vi "I2C loopback.vi"() -> ()   [LabVIEW 8.6]
uses:
  <libdir>/resource/objmgr/UeiDaq.rc
  <vilib>/UeiDaq/UeiDaqCreateI2CMasterSession.vi
  <vilib>/UeiDaq/UeiDaqConfigureTimingForMessagingIO.vi
  <vilib>/UeiDaq/UeiDaqCreateI2CSlaveSession.vi
panel:
  in  "Message Size":i32
  out "Slave Read Data String":string
  out "Master Read Data String":string
  out "Slave Read Count":i32
  out "Master Read Count":i32
  out "Command Type":u32(ring) items=["Write", "Read", "WriteRead"]
  out "Slave Tx Data":u16[](array[numeric]) format="%x"
  out "Slave Channel":i32
  out "Master Channel":i32
  in  "Stop":bool
  in  "Slave Address":i32 format="%x"
  in  "Slave Address Width":i32(ring) items=["7-bit", "10-bit"]
  in  "Bit Rate":i32(ring) items=["100kBitsPerSecond", "400kBitsPerSecond", "1MBitsPerSecond"]
  in  "TTL Level":i32(ring) items=["3.3V", "5V"]
  in  "Secure Shell?":bool
  out "Device Name":string
  in  "Resource":string
  # "I2C Loopback"
  # "Master and Slave\nCommon Configuration"
  # "Master Specific Configuration"
  # "Slave Specific Configuration"
  # "Device info"
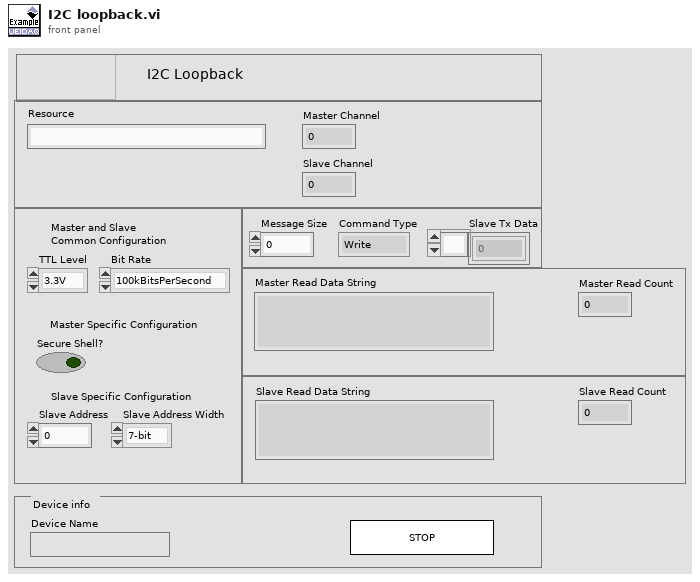
[diagram p1: front panel]
types:
  T1 = cluster{"Command":u32, "Slave Address":i32, "Slave Address Width":u32, "Number Elements to Write":i32, "Number Elements to Read":i32, "Write Data":u8[]}
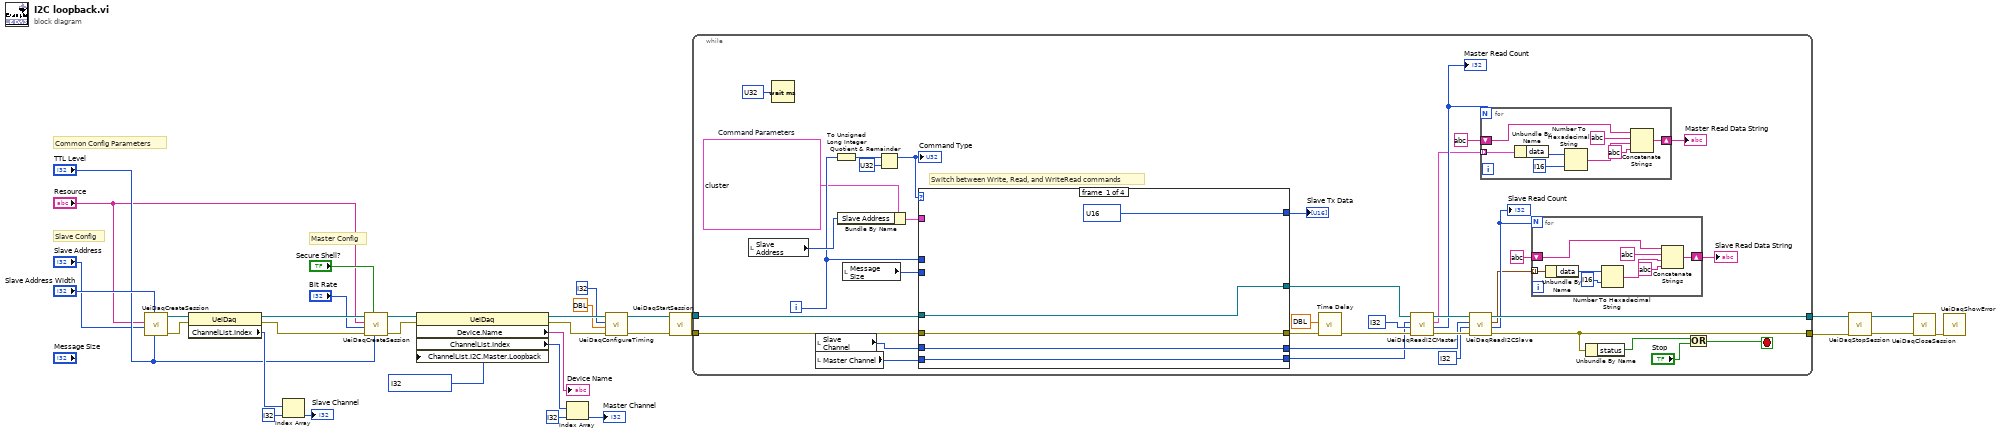
[diagram p0: block diagram]
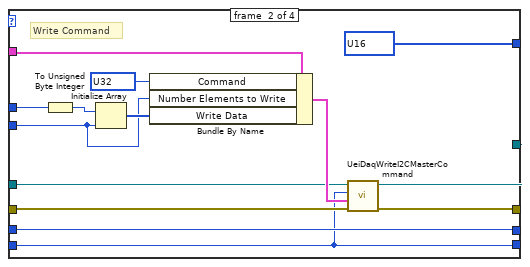
[diagram p2: hidden frame]
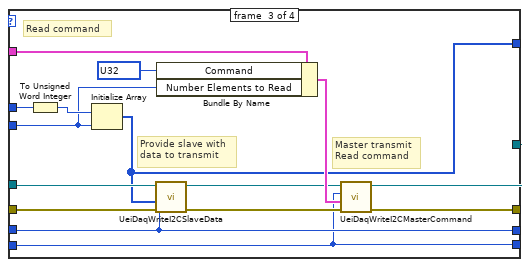
[diagram p3: hidden frame]
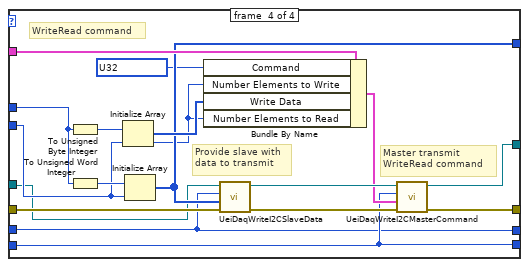
[diagram p4: hidden frame]
diagram:
  w5 = i32[] ? items=["None", "Relay", "FPGA"] ("Channel List:I2C:Master:Loopback")
  # "Master Config"
  # "Slave Config"
  # "Common Config Parameters"
  n1 = call-poly <vilib>:"UeiDaqCreateSession.vi"("TTL Level"="TTL Level", "Slave Address Width"="Slave Address Width", "Slave Address"="Slave Address", "Resource"="Resource") -> ("error out"=w22:errorcluster, "UeiDaq Refnum Out"=w25:refnum<k20>)  [unwired: 6 in]
  n2 = property class="UeiDaq"(reference=w25, error in=w22) -> (reference out=w32:refnum<k20>, error out=w31:errorcluster, "ChannelList.Index"=w27:i32[])
  n3 = Index Array(array=w27, index=i32 ?) -> (element=→"Slave Channel":i32)
  n4 = call-poly <vilib>:"UeiDaqCreateSession.vi"("TTL Level"="TTL Level", "Enable Secure Shell"="Secure Shell?", "error in (no error)"=w31, "Bit Rate"="Bit Rate", "Resource"="Resource", "UeiDaq Refnum In"=w32) -> ("error out"=w24:errorcluster, "UeiDaq Refnum Out"=w23:refnum<k20>)  [unwired: 4 in]
  n5 = property class="UeiDaq"(reference=w23, error in=w24, "ChannelList.I2C.Master.Loopback"=w5) -> (reference out=w12:refnum<k20>, error out=w11:errorcluster, "Device.Name"=→"Device Name":string, "ChannelList.Index"=w26:i32[])
  n6 = Index Array(array=w26, index=i32 ?) -> (element=→"Master Channel":i32)
  n7 = call-poly <vilib>:"UeiDaqConfigureTiming.vi"("error in (no error)"=w11, "Refresh rate"=dbl ?, "bufferSize"=i32 ?, "UeiDaq Refnum In"=w12) -> ("error out"=w16:errorcluster, "UeiDaq Refnum Out"=w15:refnum<k20>)  [unwired: 6 in]
  n8 = call <vilib>:"UeiDaqStartSession.vi"("error in (no error)"=w16, "UeiDaq Refnum In"=w15) -> ("error out"=w14:errorcluster, "UeiDaq Refnum Out"=w13:refnum<k20>)  [unwired: 8 in]
  n9 = while {
    tunnel: w14 -> [w68]
    tunnel: w13 -> [w67]
    tunnel: [w60] -> w9
    tunnel: [w51] -> w8
    i -> [w39]
    stop <- w37 stop-if-true
    w34 = T1 ?  # Command Parameters
    # "Switch between Write, Read, and WriteRead commands"
    n10 = local read "Slave Address"() -> (w55:i32)
    n11 = Wait (ms)(milliseconds to wait=u32 ?) -> ()  [unwired: 1 out]
    n12 = local read "Slave Channel"() -> (w43:i32)
    n13 = local read "Master Channel"() -> (w38:i32)
    n14 = To Unsigned Long Integer(number=w39) -> (unsigned 32bit integer=w63:u32)
    n15 = Bundle By Name(cluster=w34, "Slave Address"=w55) -> (w56:T1)
    n16 = local read "Message Size"() -> (w44:i32)
    n17 = Quotient & Remainder(x=w63, y=u32 ?) -> (x-y*floor(x/y)=w40:u32)  [unwired: 1 out]
    "Command Type" <- w40
    n18 = case shown="0" w40 {
      tunnel: w68 -> [w91 w100 w120 w134]
      tunnel: w67 -> [w90 w101 w119 w122]
      tunnel: w39 -> [_ w103 w114 w135]
      tunnel: w56 -> [_ w93 w108 w133]
      tunnel: [w90 w98 w116 w131] -> w66
      tunnel: [w91 w99 w111 w130] -> w53
      tunnel: [u16[] ? u16[] ? w107 w127] -> w62
      tunnel: w44 -> [_ w96 w106 w126]
      tunnel: w43 -> [w88 w95 w110 w123]
      tunnel: w38 -> [w87 w94 w109 w125]
      tunnel: [w88 w95 w110 w123] -> w42
      tunnel: [w87 w94 w109 w125] -> w41
      frame #0 {
      }
      frame #1 {
        w105 = u32 ? items=["Write", "Read", "WriteRead"] ("Command")
        # "Write Command"
        n19 = To Unsigned Byte Integer(number=w103) -> (unsigned 8bit integer=w92:u8)
        n20 = Initialize Array(w92, w96) -> (w104:u8[])
        n21 = Bundle By Name(cluster=w93, "Command"=w105, "Number Elements to Write"=w96, "Write Data"=w104) -> (w102:T1)
        n22 = call <vilib>:"UeiDaqWriteI2CMasterCommand.vi"("error in (no error)"=w100, "Command"=w102, "Port"=w94, "UeiDaq Refnum In"=w101) -> ("error out"=w99:errorcluster, "UeiDaq Refnum Out"=w98:refnum<k20>)  [unwired: 6 in]
      }
      frame #2 {
        w115 = u32 ? items=["Write", "Read", "WriteRead"] ("Command")
        # "Master transmit\nRead command"
        # "Provide slave with\ndata to transmit"
        # "Read command"
        n23 = To Unsigned Word Integer(number=w114) -> (unsigned 16bit integer=w113:u16)
        n24 = Initialize Array(w113, w106) -> (w107:u16[])
        n25 = call <vilib>:"UeiDaqWriteI2CSlaveData.vi"("error in (no error)"=w120, "Data"=w107, "Port"=w110, "UeiDaq Refnum In"=w119) -> ("error out"=w112:errorcluster, "UeiDaq Refnum Out"=w117:refnum<k20>)  [unwired: 5 in, 1 out]
        n26 = Bundle By Name(cluster=w108, "Command"=w115, "Number Elements to Read"=w106) -> (w118:T1)
        n27 = call <vilib>:"UeiDaqWriteI2CMasterCommand.vi"("error in (no error)"=w112, "Command"=w118, "Port"=w109, "UeiDaq Refnum In"=w117) -> ("error out"=w111:errorcluster, "UeiDaq Refnum Out"=w116:refnum<k20>)  [unwired: 6 in]
      }
      frame #3 {
        w121 = u32 ? items=["Write", "Read", "WriteRead"] ("Command")
        # "Master transmit\nWriteRead command"
        # "Provide slave with\ndata to transmit"
        # "WriteRead command"
        n28 = To Unsigned Byte Integer(number=w135) -> (unsigned 8bit integer=w124:u8)
        n29 = To Unsigned Word Integer(number=w135) -> (unsigned 16bit integer=w136:u16)
        n30 = Initialize Array(w124, w126) -> (w137:u8[])
        n31 = Initialize Array(w136, w126) -> (w127:u16[])
        n32 = Bundle By Name(cluster=w133, "Command"=w121, "Number Elements to Write"=w126, "Write Data"=w137, "Number Elements to Read"=w126) -> (w128:T1)
        n33 = call <vilib>:"UeiDaqWriteI2CSlaveData.vi"("error in (no error)"=w134, "Data"=w127, "Port"=w123, "UeiDaq Refnum In"=w122) -> ("error out"=w129:errorcluster, "UeiDaq Refnum Out"=w132:refnum<k20>)  [unwired: 5 in, 1 out]
        n34 = call <vilib>:"UeiDaqWriteI2CMasterCommand.vi"("error in (no error)"=w129, "Command"=w128, "Port"=w125, "UeiDaq Refnum In"=w132) -> ("error out"=w130:errorcluster, "UeiDaq Refnum Out"=w131:refnum<k20>)  [unwired: 6 in]
      }
    }
    "Slave Tx Data" <- w62
    n35 = call "Time Delay"("error in (no error)"=w53, "Delay Time (s)"=dbl ?) -> ("error out"=w52:errorcluster)  [unwired: 9 in]
    n36 = call <vilib>:"UeiDaqReadI2CMaster.vi"("error in (no error)"=w52, "Message count"=i32 ? ("Element count"), "Port"=w41, "UeiDaq Refnum In"=w66) -> ("error out"=w59:errorcluster, "return count"=w48:i32, "data"=w36:cluster{"stop bit":bool, "data":u8}[], "UeiDaq Refnum Out"=w61:refnum<k20>)  [unwired: 4 in]
    "Master Read Count" <- w48
    n37 = call <vilib>:"UeiDaqReadI2CSlave.vi"("error in (no error)"=w59, "Message count"=i32 ? ("Element count"), "Port"=w42, "UeiDaq Refnum In"=w61) -> ("error out"=w51:errorcluster, "return count"=w46:i32, "data"=w35:cluster{"bus code":u32, "data":u8}[], "UeiDaq Refnum Out"=w60:refnum<k20>)  [unwired: 4 in]
    "Slave Read Count" <- w46
    n38 = for {
      N: w48 -> [_]
      shift-right: [w85] -> w50
      shift-left: string ? -> [w82]
      tunnel: w36 -> [w80] mode=indexing
      n39 = Unbundle By Name(w80) -> ("data"=w79:u8)
      n40 = Number To Hexadecimal String(1:i16 ? ("width (-)"), 2:w79) -> (0:w86:string)
      n41 = Concatenate Strings(w82, string ? ("string"), w86, string ? ("string")) -> (w85:string)
    }
    "Master Read Data String" <- w50
    n42 = for {
      N: w46 -> [_]
      tunnel: w35 -> [w72] mode=indexing
      shift-right: [w78] -> w47
      shift-left: string ? -> [w75]
      n43 = Unbundle By Name(w72) -> ("data"=w71:u8)
      n44 = Number To Hexadecimal String(1:i16 ? ("width (-)"), 2:w71) -> (0:w73:string)
      n45 = Concatenate Strings(w75, string ? ("string"), w73, string ? ("string")) -> (w78:string)
    }
    "Slave Read Data String" <- w47
    n46 = Unbundle By Name(w51) -> ("status"=w58:bool)
    n47 = Or(x=w58, y="Stop") -> (x .or. y?=w37:bool)
  }
  n48 = call <vilib>:"UeiDaqStopSession.vi"("error in (no error)"=w8, "UeiDaq Refnum In"=w9) -> ("error out"=w6:errorcluster, "UeiDaq Refnum Out"=w7:refnum<k20>)  [unwired: 8 in]
  n49 = call <vilib>:"UeiDaqCloseSession.vi"("error in (no error)"=w6, "UeiDaq Refnum In"=w7) -> ("error out"=w33:errorcluster)  [unwired: 1 in, 8 out]
  n50 = call "UeiDaqShowError.vi"("error in (no error)"=w33) -> ()  [unwired: 2 in, 9 out]
